vi "Arrange Channel Group for SoftCAL.vi"(0 "Channel Group":T1, 5 "Channel Type":enum16{"Voltage", "Thermocouple"}(ring), 7 "Thermocouple Type":u16) -> (4 "SoftCAL Channel Config":T3(array[cluster]))   [LabVIEW 2019]
uses:
  Type Defs and Controls/Channel Cluster.ctl
  Type Defs and Controls/Channel Config.ctl
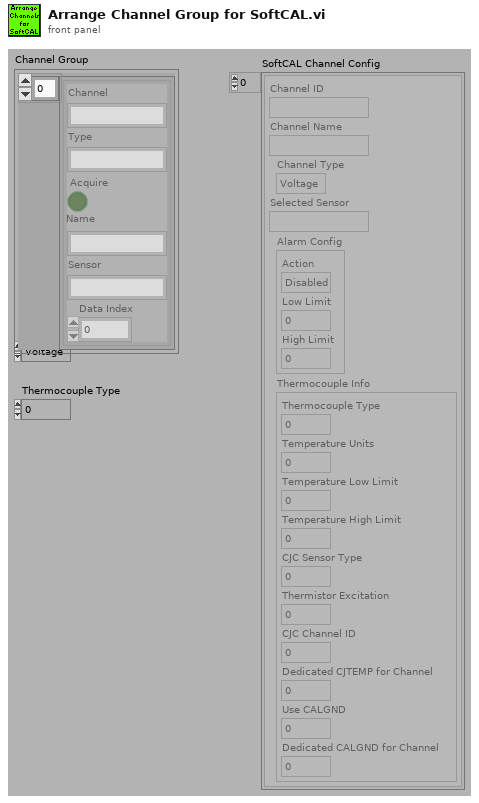
[diagram p1: front panel]
types:
  T1 = typedef "Channel Cluster.ctl" = cluster{"Channels":T2[]}
  T2 = typedef "Channel Config.ctl" = cluster{"Channel":string, "Type":string, "Acquire":bool, "Name":string, "Sensor":string, "Data Index":u32}
  T3 = cluster{"Channel ID":string, "Channel Name":string, "Channel Type":enum16{"Voltage", "Thermocouple"}, "Selected Sensor":string, "Alarm Config":cluster{"Action":enum16{"Disabled", "Display On-Screen Warning", "Shutdown System"}, "Low Limit":dbl, "High Limit":dbl}, "Thermocouple Info":cluster{"Thermocouple Type":u16, "Temperature Units":u16, "Temperature Low Limit":sgl, "Temperature High Limit":sgl, "CJC Sensor Type":u16, "Thermistor Excitation":u16, "CJC Channel ID":u16, "Dedicated CJTEMP for Channel":u16, "Use CALGND":u16, "Dedicated CALGND for Channel":u16}}[]
  T4 = cluster{"Channel ID":string, "Channel Name":string, "Channel Type":enum16{"Voltage", "Thermocouple"}, "Selected Sensor":string, "Alarm Config":cluster{"Action":enum16{"Disabled", "Display On-Screen Warning", "Shutdown System"}, "Low Limit":dbl, "High Limit":dbl}, "Thermocouple Info":cluster{"Thermocouple Type":u16, "Temperature Units":u16, "Temperature Low Limit":i32, "Temperature High Limit":i32, "CJC Sensor Type":u16, "Thermistor Excitation":u16, "CJC Channel ID":u16, "Dedicated CJTEMP for Channel":u16, "Use CALGND":u16, "Dedicated CALGND for Channel":u16}}
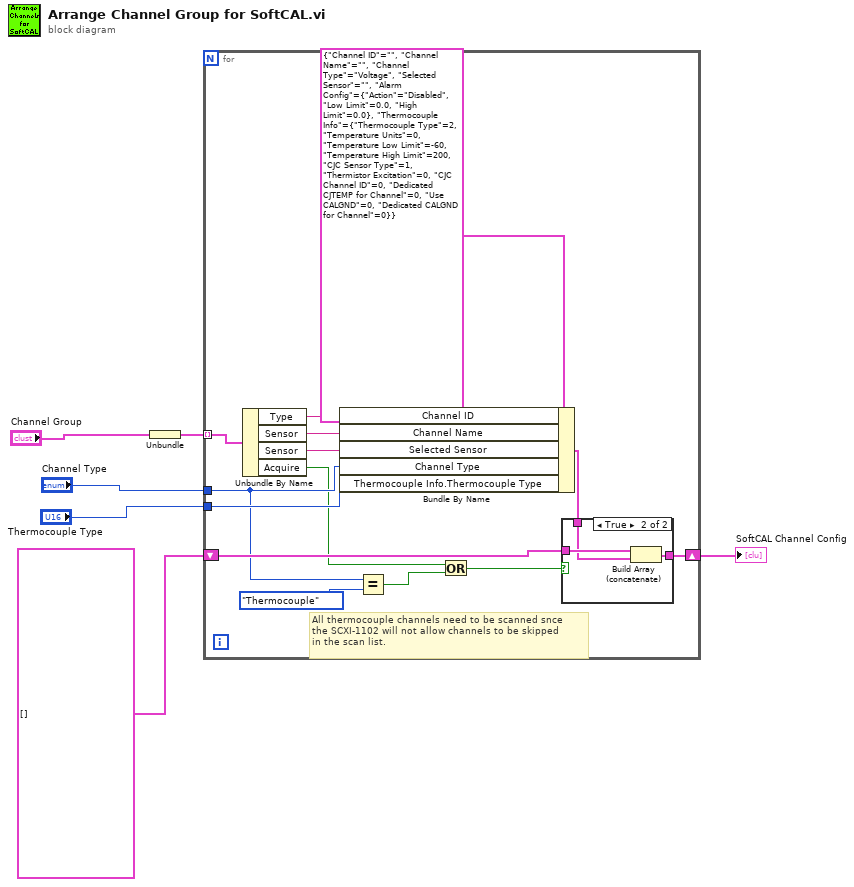
[diagram p0: block diagram]
diagram:
  n1 = Unbundle("Channel Group") -> ("Channels"=w4:T2[])
  n2 = for {
    tunnel: w4 -> [w19] mode=indexing
    tunnel: "Channel Type" -> [w11]
    tunnel: "Thermocouple Type" -> [w12]
    shift-right: [w13] -> w1
    shift-left: T3 [] ("SoftCAL Channel Config") -> [w15]
    # "All thermocouple channels need to be scanned snce\nthe SCXI-1102 will not allow channels to be skipped\nin the scan list."
    n3 = Unbundle By Name(w19) -> ("Type"=w18:string, "Sensor"=w16:string, "Sensor"=w17:string, "Acquire"=w9:bool)
    n4 = Bundle By Name(cluster=T4 {"Channel ID"="", "Channel Name"="", "Channel Type"=enum."Voltage", "Selected Sensor"="", "Alarm Config"={"Action"=enum."Disabled", "Low Limit"=0.0, "High Limit"=0.0}, "Thermocouple Info"={"Thermocouple Type"=2, "Temperature Units"=0, "Temperature Low Limit"=-60, "Temperature High Limit"=200, "CJC Sensor Type"=1, "Thermistor Excitation"=0, "CJC Channel ID"=0, "Dedicated CJTEMP for Channel"=0, "Use CALGND"=0, "Dedicated CALGND for Channel"=0}} ("Channel Config"), "Channel ID"=w18, "Channel Name"=w16, "Selected Sensor"=w17, "Channel Type"=w11, "Thermocouple Info.Thermocouple Type"=w12) -> (w14:T4)
    n5 = Equal?(x=w11, y=enum16{"Voltage", "Thermocouple"}."Thermocouple") -> (x = y?=w8:bool)
    n6 = Or(x=w9, y=w8) -> (x .or. y?=w7:bool)
    n7 = case shown="True" w7 {
      tunnel: w15 -> [w21 w24]
      tunnel: w14 -> [_ w23]
      tunnel: [w21 w22] -> w13
      frame False {
      }
      frame True {
        n8 = Build Array (concatenate)(w24, w23) -> (w22:T3)
      }
    }
  }
  "SoftCAL Channel Config" <- w1
